vi "Test peseli.vi"() -> ()   [LabVIEW 2023]
panel:
  out "WYJSCIE":T1
  in  "stop":bool
  in  "WEJSCIE":T2
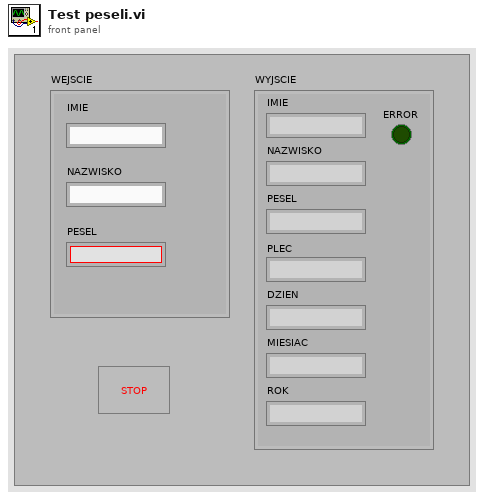
[diagram p1: front panel]
types:
  T1 = cluster{"NAZWISKO":string, "IMIE":string, "PESEL":string, "ERROR":bool, "DZIEN":string, "MIESIAC":string, "ROK":string, "PLEC":string}
  T2 = cluster{"NAZWISKO":string, "IMIE":string, "PESEL":string}
  T3 = cluster{"NAZWISKO":string, "IMIE":string, "PESEL":string, bool, string, string, string, string}
  T4 = cluster{string, string, "PESEL":string, bool, string, string, string, string}
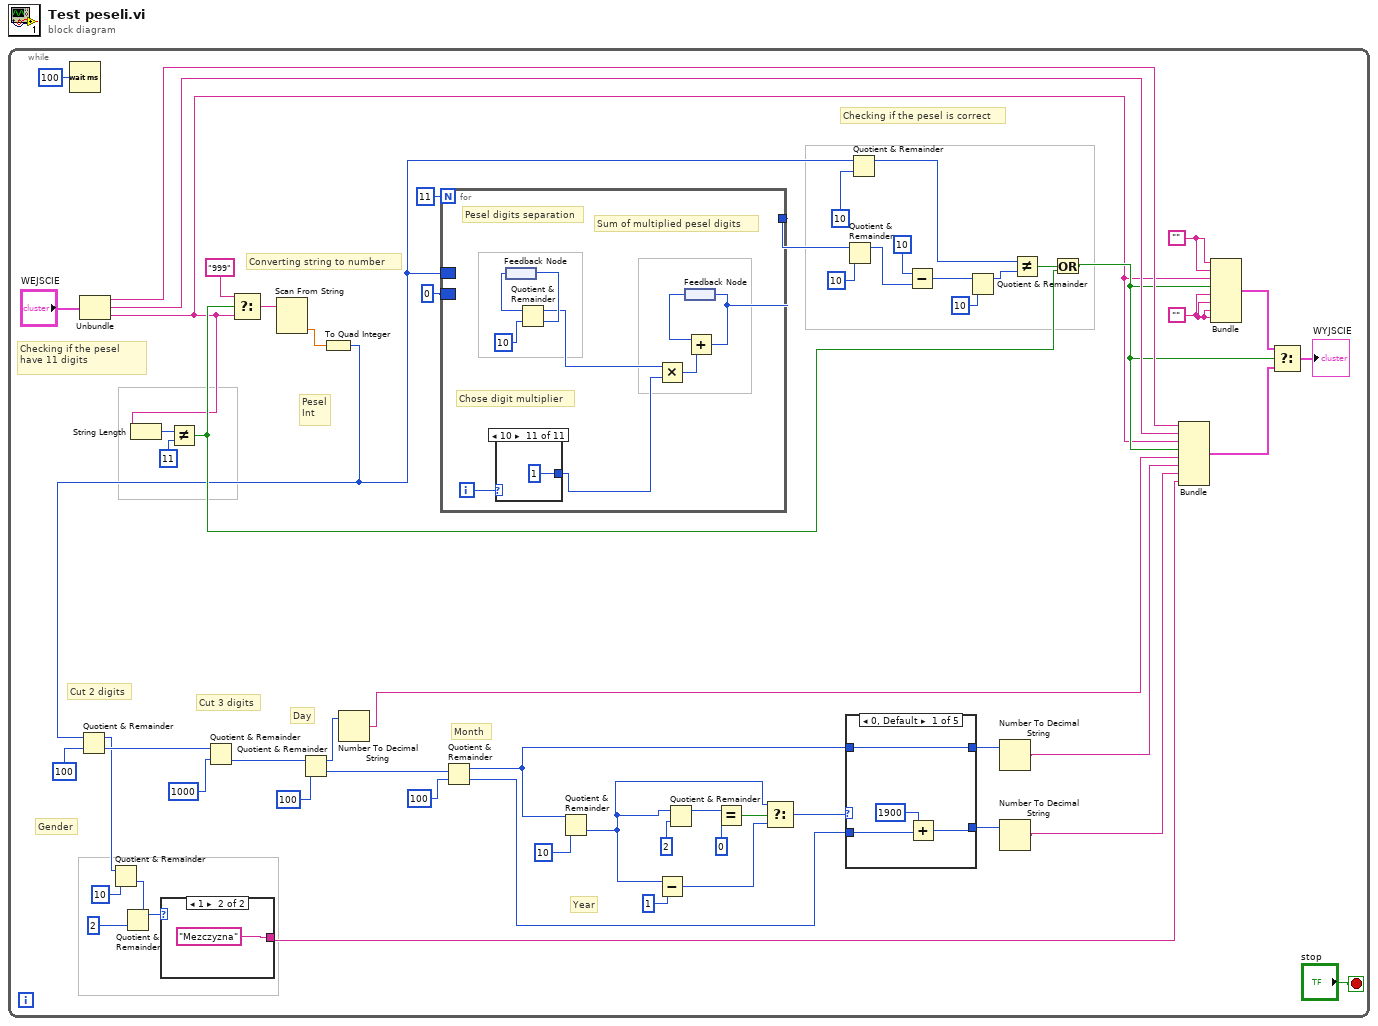
[diagram p0: block diagram]
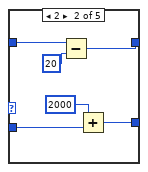
[diagram p2: hidden frame]
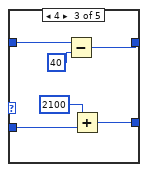
[diagram p3: hidden frame]
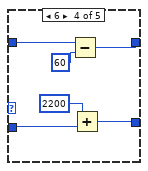
[diagram p4: hidden frame]
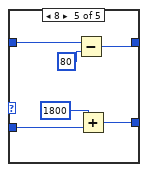
[diagram p5: hidden frame]
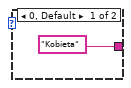
[diagram p6: hidden frame]
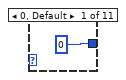
[diagram p7: hidden frame]
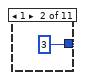
[diagram p8: hidden frame]
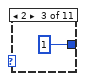
[diagram p9: hidden frame]
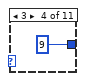
[diagram p10: hidden frame]
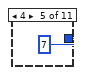
[diagram p11: hidden frame]
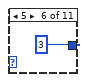
[diagram p12: hidden frame]
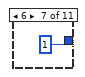
[diagram p13: hidden frame]
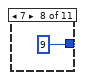
[diagram p14: hidden frame]
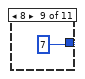
[diagram p15: hidden frame]
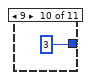
[diagram p16: hidden frame]
diagram:
  n1 = while {
    stop <- "stop" stop-if-true
    w7 = ""
    w8 = ""
    # "Pesel\nInt"
    # "Checking if the pesel \nhave 11 digits"
    # "Year"
    # "Cut 2 digits"
    # "Cut 3 digits"
    # "Month"
    # "Day"
    # "Gender"
    # "Converting string to number"
    # "Checking if the pesel is correct"
    n2 = Wait (ms)(milliseconds to wait=100) -> ()  [unwired: 1 out]
    n3 = Unbundle("WEJSCIE") -> ("NAZWISKO"=w18:string, "IMIE"=w17:string, "PESEL"=w4:string)
    n4 = String Length(string=w4) -> (length=w41:i32)
    n5 = Not Equal?(x=w41, y=11) -> (x != y?=w6:bool)
    n6 = Select(t="999", s=w6, f=w4) -> (s? t:f=w5:string)
    n7 = Scan From String(input string=w5) -> (output 1=w29:dbl)  [unwired: 4 in, 3 out]
    n8 = To Quad Integer(1:w29) -> (0:w2:i64)
    n9 = Quotient & Remainder(x=w2, y=100) -> (x-y*floor(x/y)=w23:i64, floor(x/y)=w48:i64)
    n10 = Quotient & Remainder(x=w23, y=10) -> (floor(x/y)=w22:i64)  [unwired: 1 out]
    n11 = Quotient & Remainder(x=w22, y=2) -> (x-y*floor(x/y)=w49:i64)  [unwired: 1 out]
    n12 = case shown="1" w49 {
      tunnel: ["Kobieta" "Mezczyzna"] -> w11
      frame 0, Default {
      }
      frame 1 {
      }
    }
    n13 = Quotient & Remainder(x=w48, y=1000) -> (floor(x/y)=w46:i64)  [unwired: 1 out]
    n14 = Quotient & Remainder(x=w46, y=100) -> (x-y*floor(x/y)=w21:i64, floor(x/y)=w44:i64)
    n15 = Number To Decimal String(number=w21) -> (decimal integer string=w14:string)  [unwired: 1 in]
    n16 = for {
      N: 11 -> [_]
      tunnel: [w98] -> w57
      border: 0 -> [_]
      border: w2 -> [_]
      i -> [w96]
      # "Sum of multiplied pesel digits"
      # "Chose digit multiplier"
      # "Pesel digits separation"
      n17 = case shown="10" w96 {
        tunnel: [0 3 1 9 7 3 1 9 7 3 1] -> w92
        frame 0, Default {
        }
        frame 1 {
        }
        frame 2 {
        }
        frame 3 {
        }
        frame 4 {
        }
        frame 5 {
        }
        frame 6 {
        }
        frame 7 {
        }
        frame 8 {
        }
        frame 9 {
        }
        frame 10 {
        }
      }
      n18 = feedback #1() -> (w94:i64)
      n19 = Quotient & Remainder(x=w94, y=10) -> (x-y*floor(x/y)=w95:i64, floor(x/y)=w97:i64)
      n20 = feedback-in #1(w97) -> ()
      n21 = Multiply(x=w95, y=w92) -> (x*y=w99:i64)
      n22 = feedback #2() -> (w100:i64)
      n23 = Add(x=w100, y=w99) -> (x+y=w98:i64)
      n24 = feedback-in #2(w98) -> ()
    }
    n25 = Quotient & Remainder(x=w44, y=100) -> (x-y*floor(x/y)=w30:i64, floor(x/y)=w33:i64)
    n26 = Quotient & Remainder(x=w30, y=10) -> (floor(x/y)=w31:i64)  [unwired: 1 out]
    n27 = Subtract(x=w31, y=1) -> (x-y=w35:i64)
    n28 = Quotient & Remainder(x=w31, y=2) -> (x-y*floor(x/y)=w39:i64)  [unwired: 1 out]
    n29 = Equal?(x=w39, y=0) -> (x = y?=w37:bool)
    n30 = Select(t=w31, s=w37, f=w35) -> (s? t:f=w34:i64)
    n31 = Quotient & Remainder(x=w57, y=10) -> (x-y*floor(x/y)=w54:i64)  [unwired: 1 out]
    n32 = case shown="0, Default" w34 {
      tunnel: w33 -> [w63 w70 w76 w81 w87]
      tunnel: [w64 w69 w75 w82 w88] -> w19
      tunnel: w30 -> [w62 w67 w72 w78 w84]
      tunnel: [w62 w68 w73 w79 w85] -> w20
      frame 0, Default {
        n33 = Add(x=1900, y=w63) -> (x+y=w64:i64)
      }
      frame 2 {
        n34 = Subtract(x=w67, y=20) -> (x-y=w68:i64)
        n35 = Add(x=2000, y=w70) -> (x+y=w69:i64)
      }
      frame 4 {
        n36 = Subtract(x=w72, y=40) -> (x-y=w73:i64)
        n37 = Add(x=2100, y=w76) -> (x+y=w75:i64)
      }
      frame 6 {
        n38 = Subtract(x=w78, y=60) -> (x-y=w79:i64)
        n39 = Add(x=2200, y=w81) -> (x+y=w82:i64)
      }
      frame 8 {
        n40 = Subtract(x=w84, y=80) -> (x-y=w85:i64)
        n41 = Add(x=1800, y=w87) -> (x+y=w88:i64)
      }
    }
    n42 = Quotient & Remainder(x=w2, y=10) -> (x-y*floor(x/y)=w52:i64)  [unwired: 1 out]
    n43 = Subtract(x=10, y=w54) -> (x-y=w27:i64)
    n44 = Quotient & Remainder(x=w27, y=10) -> (x-y*floor(x/y)=w26:i64)  [unwired: 1 out]
    n45 = Number To Decimal String(number=w20) -> (decimal integer string=w15:string)  [unwired: 1 in]
    n46 = Number To Decimal String(number=w19) -> (decimal integer string=w16:string)  [unwired: 1 in]
    n47 = Not Equal?(x=w52, y=w26) -> (x != y?=w25:bool)
    n48 = Or(x=w25, y=w6) -> (x .or. y?=w9:bool)
    n49 = Bundle("NAZWISKO"=w18, "IMIE"=w17, "PESEL"=w4, w9, w14, w15, w16, w11) -> (w12:T3)  [unwired: 1 in]
    n50 = Bundle(w7, w7, "PESEL"=w4, w9, w8, w8, w8, w8) -> (w10:T4)  [unwired: 1 in]
    n51 = Select(t=w10, s=w9, f=w12) -> (s? t:f=→"WYJSCIE":T3)
  }
